vi "Start Config.vi"(8 "error in":errorcluster, 11 "nPAS in":refnum<class "nPAS.lvclass">) -> (0 "error out":errorcluster, 3 "nPAS out":refnum<class "nPAS.lvclass">)   [LabVIEW 2015, in "nPAS.lvclass"]
doc: "Perform configuration of cells and data classes as well as switching and anything else that might not fit into the other config VIs. This VI can be used to set up a single cell with the default PAS Data Class, PAS Cell class, and a speaker switch setting of firing every 5 minutes for 1 second."
uses:
  nPAS.lvclass
  Session/Raw FPGA/FPGA Session.lvclass
  nPAS.lvclass/nPAS.ctl
  Session/Raw FPGA/FPGA Session.lvclass/FPGA Session.ctl
  Session/Raw FPGA/Read FPGA Ref.vi
  <vilib>/Utility/error.llb/Error Cluster From Error Code.vi
  <vilib>/rvi/errors/niLvFpgaAdjustHostInterfaceError.vi
  FPGA Ref.ctl
  <vilib>/rvi/interface/nirviReadWriteControl/nirviReadWriteControl.xnode
  FPGA Bitfiles/NickIO.lvbitx
  <userlib>/_Session Fwk/Session - Root.lvclass
  NiFpgaLv.dll
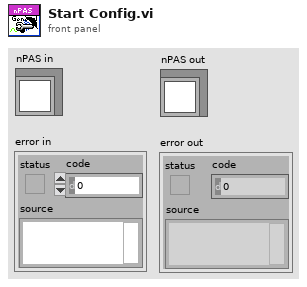
[diagram p1: front panel]
types:
  T1 = typedef "Session - Root.lvclass/Session Handle.ctl" = refnum<data-value>
  T2 = typedef "FPGA Ref.ctl" = refnum<k20>
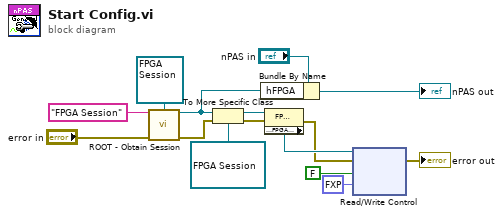
[diagram p0: block diagram]
diagram:
  n1 = call <userlib>:"ROOT - Obtain Session.vi"("Session Name ()"="FPGA Session", "OBJ - Session"=refnum<class "FPGA Session.lvclass"> refnum ("FPGA Session.lvclass"), "error in (no error)"="error in") -> ("Session Handle"=w3:T1, "error out"=w9:errorcluster)  [unwired: 10 in, 1 out]
  n2 = To More Specific Class(target class=refnum<data-value> refnum ("hFPGA"), reference=w3, error in=w9) -> (specific class reference=w8:refnum<data-value>, error out=w7:errorcluster)
  n3 = Bundle By Name(cluster="nPAS in", "hFPGA"=w3) -> (→"nPAS out":refnum<class "nPAS.lvclass">)
  n4 = property class="FPGA Session"(reference=w8, error in=w7) -> (error out=w13:errorcluster, "Accessors:FPGA Ref"=w14:T2)  [unwired: 1 out]
  n5 = xnode "Read/Write Control"("FPGA VI Reference In"=w14, "error in"=w13, "Stop"=FALSE, "pDC"=fxp<+,32,0> 0.5 ("Duty Cycle")) -> ("error out"=→"error out":errorcluster)  [unwired: 1 out]
